vi "Read Skillbook.vi"(8 "error in (no error)":errorcluster, 11 "Tactic in":refnum<class "Tactic.lvclass">) -> (0 "error out":errorcluster, 2 "Skillbook":refnum<class "Skillbook.lvclass">, 3 "Tactic out":refnum<class "Tactic.lvclass">)   [LabVIEW 2023, in "Tactic.lvclass"]
uses:
  Tactic.lvclass
  Skillbook_class/Skillbook.lvclass
  Tactic.lvclass/Tactic.ctl
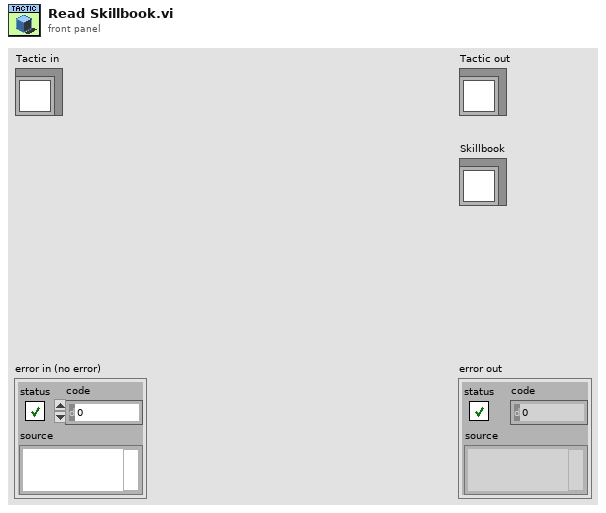
[diagram p1: front panel]
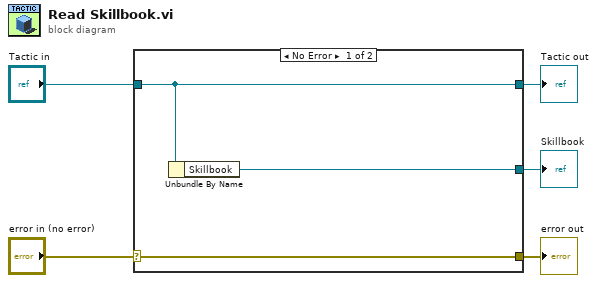
[diagram p0: block diagram]
diagram:
  n1 = case shown="No Error" "error in (no error)" {
    selector: "error in (no error)" -> [w8 w9]
    tunnel: [w8 w9] -> w4
    tunnel: [w7 w10] -> w2
    tunnel: "Tactic in" -> [w7 w10]
    tunnel: [w6 _] -> w1
    frame No Error {
      n2 = Unbundle By Name(w7) -> ("Skillbook"=w6:refnum<class "Skillbook.lvclass">)
    }
    frame Error {
    }
  }
  "error out" <- w4
  "Tactic out" <- w2
  "Skillbook" <- w1
